vi "PLTS.vi"() -> ()   [LabVIEW 2011]
panel:
  out "ImportFile":variant
  in  "ppView":variant
  in  "ppDoc":variant
  in  "PLTS.IPLTSview":refnum<k7>
  in  "PLTS.IPLTSDoc":refnum<k7>
  in  "Path":path=path "D:/TX3.s4p"
  in  "Analysis Type":T1(ring)
  in  "PLTS.IPLTSApplication":refnum<k7>
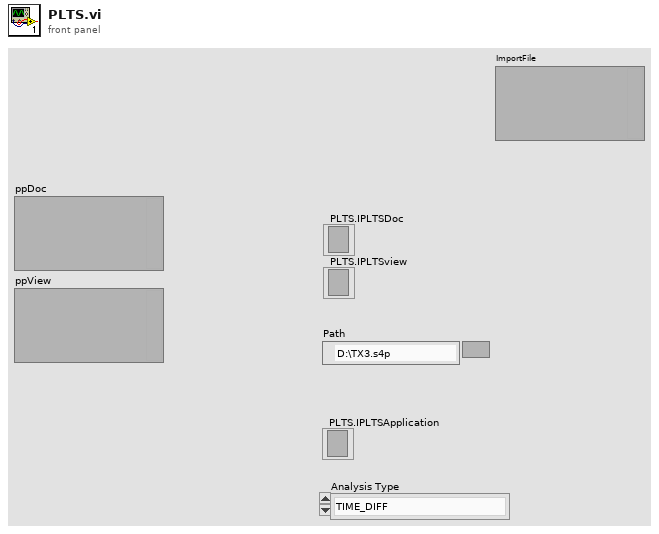
[diagram p1: front panel]
types:
  T1 = enum16{"TIME_DIFF", "TIME_SNGL", "FREQ_BAL", "FRE_SNGL", "EYE_DIFF", "EYE_SNGL"}
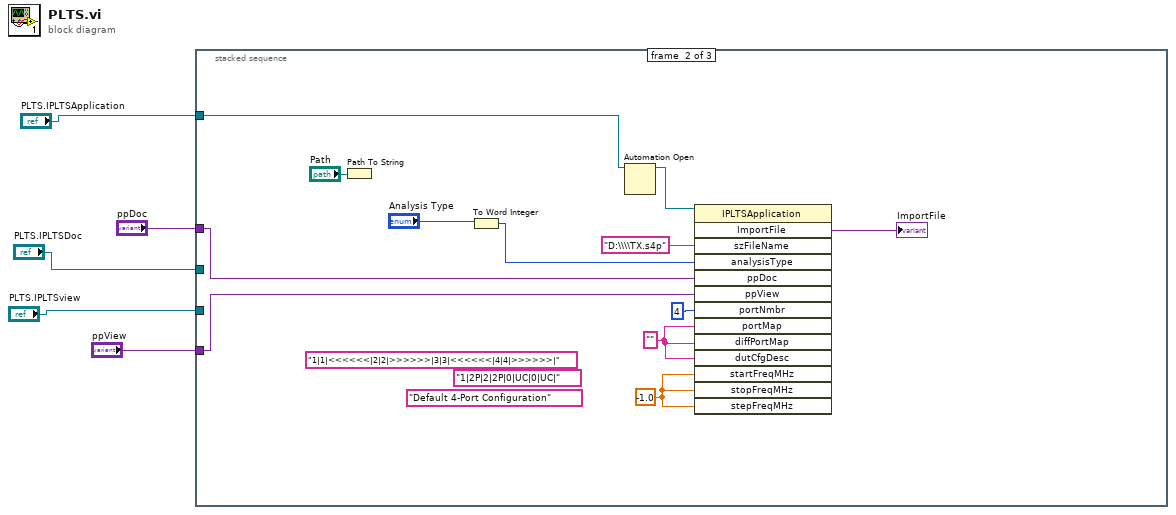
[diagram p0: block diagram]
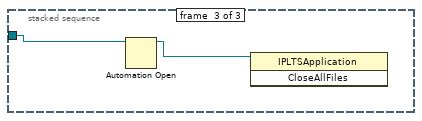
[diagram p3: hidden frame]
diagram:
  n1 = stacked-sequence {
    tunnel: "PLTS.IPLTSApplication" -> [_ w12 w19]
    tunnel: "PLTS.IPLTSDoc" -> [_ _ _]
    tunnel: "PLTS.IPLTSview" -> [_ _ _]
    tunnel: "ppDoc" -> [_ w9 _]
    tunnel: "ppView" -> [_ w8 _]
    frame #0 {
    }
    frame #1 {
      w11 = "" ("portMap")
      (unwired) "1|1|<<<<<<|2|2|>>>>>>|3|3|<<<<<<|4|4|>>>>>>|" ("dutCfgDesc")
      (unwired) "1|2P|2|2P|0|UC|0|UC|" ("diffPortMap")
      (unwired) "Default 4-Port Configuration" ("dutCfgDesc")
      w16 = -1.0 ("startFreqMHz")
      n2 = Path To String(path="Path") -> ()  [unwired: 1 out]
      n3 = To Word Integer(number="Analysis Type") -> (16bit integer=w14:i16)
      n4 = Automation Open(Automation Refnum=w12) -> (Automation Refnum=w10:refnum<k7>)  [unwired: 3 in, 1 out]
      n5 = invoke class="IPLTSApplication" method="ImportFile"(reference=w10, "szFileName"="D:\\\\TX.s4p", "analysisType"=w14, "ppDoc"=w9, "ppView"=w8, "portNmbr"=i16 4, "portMap"=w11, "diffPortMap"=w11, "dutCfgDesc"=w11, "startFreqMHz"=w16, "stopFreqMHz"=w16, "stepFreqMHz"=w16) -> ("ImportFile"=→"ImportFile":variant)  [unwired: 2 in, 13 out]
    }
    frame #2 {
      n6 = Automation Open(Automation Refnum=w19) -> (Automation Refnum=w18:refnum<k7>)  [unwired: 3 in, 1 out]
      n7 = invoke class="IPLTSApplication" method="CloseAllFiles"(reference=w18) -> ()  [unwired: 2 in, 3 out]
    }
  }
